vi "Add Component Dependencies.vi"(8 "error in (no error)":errorcluster, 11 "Device Item Ref in":T1 format="%.0x") -> (0 "error out":errorcluster, 2 "component names":string[](array[string]), 3 "Device Ref out":T1 format="%.0x")   [LabVIEW 2017, in "DSF System Explorer.lvlib"]
uses:
  DSF System Explorer.lvlib
  <vilib>/NI Veristand/Custom Device API/Custom Device Item Ref.ctl
  <vilib>/NI Veristand/Custom Device API/Set Item Property (Path).vi
  <vilib>/NI Veristand/Custom Device API/Custom Device API.lvlib
  Shared/DSF Shared.lvlib
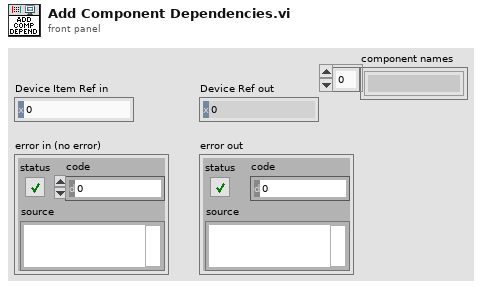
[diagram p1: front panel]
types:
  T1 = typedef "Custom Device API.lvlib/Custom Device Item Ref.ctl" = u64
  T2 = typedef "Custom Device API.lvlib/Custom Device Target Type.ctl" = enum16{"PharLap", "VxWorks", "Windows", "Linux_32_ARM", "Linux_x64"}
  T3 = typedef "Custom Device API.lvlib/Custom Device File Dependency.ctl" = cluster{"Source":T4, "RT Destination":path, "ForceDownload?":bool, "SupportedTarget":T6, "Version":string}
  T4 = typedef "Custom Device API.lvlib/Path Specification.ctl" = cluster{"Path":path, "Type":T5}
  T5 = typedef "Custom Device API.lvlib/Path Type.ctl" = enum16{"Absolute", "To Base", "To Common Data Dir", "To Application Data Dir"}
  T6 = typedef "Custom Device API.lvlib/Custom Device Supported Target.ctl" = enum16{"All", "PharLap", "VxWorks", "Windows", "Linux_32_ARM", "Linux_x64", "PharLap & Windows", "PharLap & VxWorks", "VxWorks & Windows"}
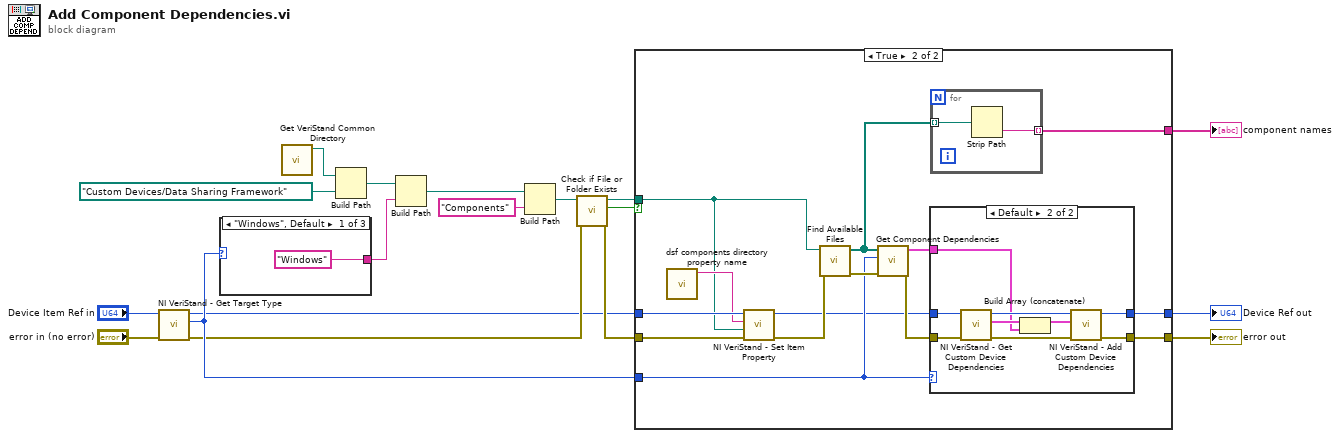
[diagram p0: block diagram]
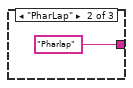
[diagram p4: hidden frame]
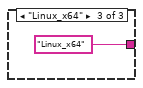
[diagram p5: hidden frame]
diagram:
  n1 = call <vilib>:"NI VeriStand - Get Target Type.vi"("error in (no error)"="error in (no error)", "Item Ref in"="Device Item Ref in") -> ("error out"=w6:errorcluster, "Target Type"=w10:T2, "Item Ref out"=w4:T1)  [unwired: 7 in]
  n2 = case shown="\"Windows\", Default" w10 {
    tunnel: ["Windows" "Pharlap" "Linux_x64"] -> w12
    frame "Windows", Default {
    }
    frame "PharLap" {
    }
    frame "Linux_x64" {
    }
  }
  n3 = call "Get VeriStand Common Directory.vi"() -> ("common directory"=w15:path)  [unwired: 11 in]
  n4 = Build Path(base path=w15, name or relative path=path "Custom Devices/Data Sharing Framework") -> (appended path=w17:path)
  n5 = Build Path(base path=w17, name or relative path=w12) -> (appended path=w13:path)
  n6 = Build Path(base path=w13, name or relative path="Components") -> (appended path=w2:path)
  n7 = call <vilib>:"Check if File or Folder Exists.vi"("error in (no error)"=w6, "path"=w2) -> ("error out"=w5:errorcluster, "file or folder exists?"=w3:bool, "dup path"=w7:path)  [unwired: 7 in]
  n8 = case shown="True" w3 {
    tunnel: [w22 w37] -> w18
    tunnel: [w23 w36] -> w1
    tunnel: [_ w31] -> w11
    tunnel: w4 -> [w22 w30]
    tunnel: w10 -> [_ w29]
    tunnel: w7 -> [_ w25]
    tunnel: w5 -> [w23 w24]
    frame False {
    }
    frame True {
      n9 = call "dsf components directory property name.vi"() -> ("components directory property name"=w26:string)  [unwired: 11 in]
      n10 = call-poly <vilib>:"NI VeriStand - Set Item Property.vi"("error in (no error)"=w24, "Value"=w25, "Property Name"=w26, "Item Ref in"=w30) -> ("error out"=w28:errorcluster, "Item Ref out"=w27:T1)  [unwired: 5 in, 1 out]
      n11 = call "Find Available Files.vi"("error in (no error)"=w28, "components directory"=w25) -> ("error out"=w33:errorcluster, "paths"=w32:path[])  [unwired: 8 in]
      n12 = call "Get Component Dependencies.vi"("error in (no error)"=w33, "Target Type"=w29, "component paths"=w32) -> ("error out"=w35:errorcluster, "component dependencies"=w34:T3[])  [unwired: 7 in]
      n13 = case shown="Default" w29 {
        tunnel: w34 -> [_ w43]
        tunnel: w35 -> [w41 w49]
        tunnel: w27 -> [w40 w50]
        tunnel: [w41 w44] -> w36
        tunnel: [w40 w42] -> w37
        frame "Windows" {
          # "Don't add dependencies for Windows."
        }
        frame Default {
          n14 = call <vilib>:"NI VeriStand - Get Custom Device Dependencies.vi"("error in (no error)"=w49, "Device Ref in"=w50) -> ("error out"=w47:errorcluster, "Dependencies"=w48:T3[], "Device Ref out"=w45:T1)  [unwired: 7 in]
          n15 = Build Array (concatenate)(w48, w43) -> (w46:T3[])
          n16 = call <vilib>:"NI VeriStand - Add Custom Device Dependencies.vi"("error in (no error)"=w47, "Dependencies"=w46, "Device Ref in"=w45) -> ("error out"=w44:errorcluster, "Device Ref out"=w42:T1)  [unwired: 7 in]
        }
      }
      n17 = for {
        tunnel: w32 -> [w39] mode=indexing
        tunnel: [w38] -> w31 mode=indexing
        n18 = Strip Path(path=w39) -> (name=w38:string)  [unwired: 1 out]
      }
    }
  }
  "Device Ref out" <- w18
  "error out" <- w1
  "component names" <- w11
